vi "Target_new.vi"() -> ()   [LabVIEW 2013]
uses:
  <vilib>/Platform/TimedLoop/XDataNode/timing_clust.ctl
  <vilib>/Platform/TimedLoop/XDataNode/nitl_modes.ctl
  <vilib>/Platform/TimedLoop/XDataNode/wakeup.ctl
  <vilib>/rvi/Emulation/niFpgaSctlEmulationGetInTimedLoop.vi
  <vilib>/rvi/Emulation/niFpgaEmulationReportErrorSimple.vi
  <vilib>/rvi/Emulation/niFpgaGetClockAttributes.vi
  <vilib>/rvi/Emulation/niFpgaCriticalErrorInLSC.vi
  <vilib>/rvi/interface/RandomDataEmulation/nirviRandomDataFPGAFIFO.vi
  <vilib>/rvi/interface/RandomDataEmulation/niFpgaRandomDataHandleErrors.vi
  <vilib>/rvi/DataTransferAndStorage/Container/Common/niFpgaContainerGetUniqueNameForEmu.vi
  <vilib>/rvi/Memory/Memory_Emulation/niFpgaMemoryEmulationReadFromVariant.vi
  <vilib>/rvi/Memory/Memory_Emulation/niFpgaMemoryFastEmulationDramWriteAndRequestData.vi
  <vilib>/rvi/Memory/Memory_Emulation/niFpgaMemoryEmulationDramWriteAndRequestData.vi
  <vilib>/rvi/Memory/Memory_Emulation/niFpgaMemoryEmulationWriteToVariant.vi
  <vilib>/Platform/TimedLoop/XDataNode/XDataNode.xnode
  <vilib>/rvi/DataTransferAndStorage/Container/XNode/niFpgaContainer.xnode
  <vilib>/rvi/interface/RandomDataEmulation/nirviRandomDataFpgaReadWriteTemplate.vi
  <vilib>/rvi/Memory/Memory_Emulation/niFpgaMemoryEmulationDramRetrieveData.vi
  <vilib>/Platform/TimedLoop/XDataNode/XDNodeRunTimeDep.lvlib
panel:
  out "Записали FIFO":bool
  in  "Кон_адр":u32
  in  "FIFO":bool
  in  "Address":u32
  out "Data":u8
  in  "4":u8=4
  in  "2":u8=2
  out "Number of Elements to Write":u32
  in  "Чтение DRAM":bool
  in  "Нач_адр":u32
  in  "HOST":bool
  in  "D-0":u32
  in  "Запись в DRAM":bool
  in  "Стоп":bool
  in  "2097152":u32=2146304
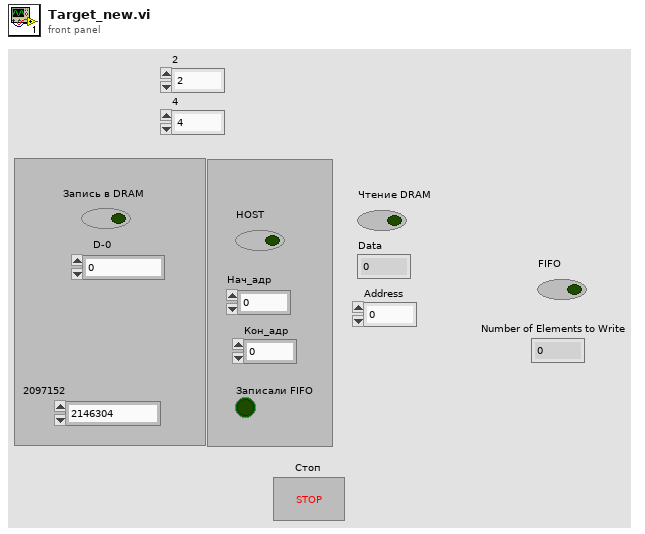
[diagram p1: front panel]
types:
  T1 = typedef "XDNodeRunTimeDep.lvlib/timing_clust.ctl" = cluster{"Expected End [f-1]":u64, "Actual End [f-1]":u64, "Finished Late? [f-1]":bool, "Expected End [i-1]":u64, "Actual End [i-1]":u64, "Finished Late? [i-1]":bool, "Expected Start [i]":u64, "Actual Start [i]":u64, "Expected Start [f]":u64, "Actual Start [f]":u64, "Source Name":string, "Structure Name":string, "Period":i64, "Deadline":i64, "Offset":i64, "Start":i64, "Priority":i32, "Timeout":i32, "Mode":T2, "Wakeup Reason":T3, "Error":errorcluster, "Source Type":string, "Secondary Source Type":string, "Global End Time":u64, "Global Start Time":u64, "Frame Duration":u64, "Iteration Duration":u64, "Assigned CPU":i32, "I/O Scan Engine Mode":u32}
  T2 = typedef "XDNodeRunTimeDep.lvlib/nitl_modes.ctl" = enum32{"No Change", "Process missed periods, maintain original phase", "Discard missed periods, maintain original phase", "Process missed periods, ignore original phase", "Discard missed periods, ignore original phase"}
  T3 = typedef "XDNodeRunTimeDep.lvlib/wakeup.ctl" = enum32{"Normal", "Aborted", "Asynchronous wakeup", "Timing source error", "Timed loop error", "Timeout"}
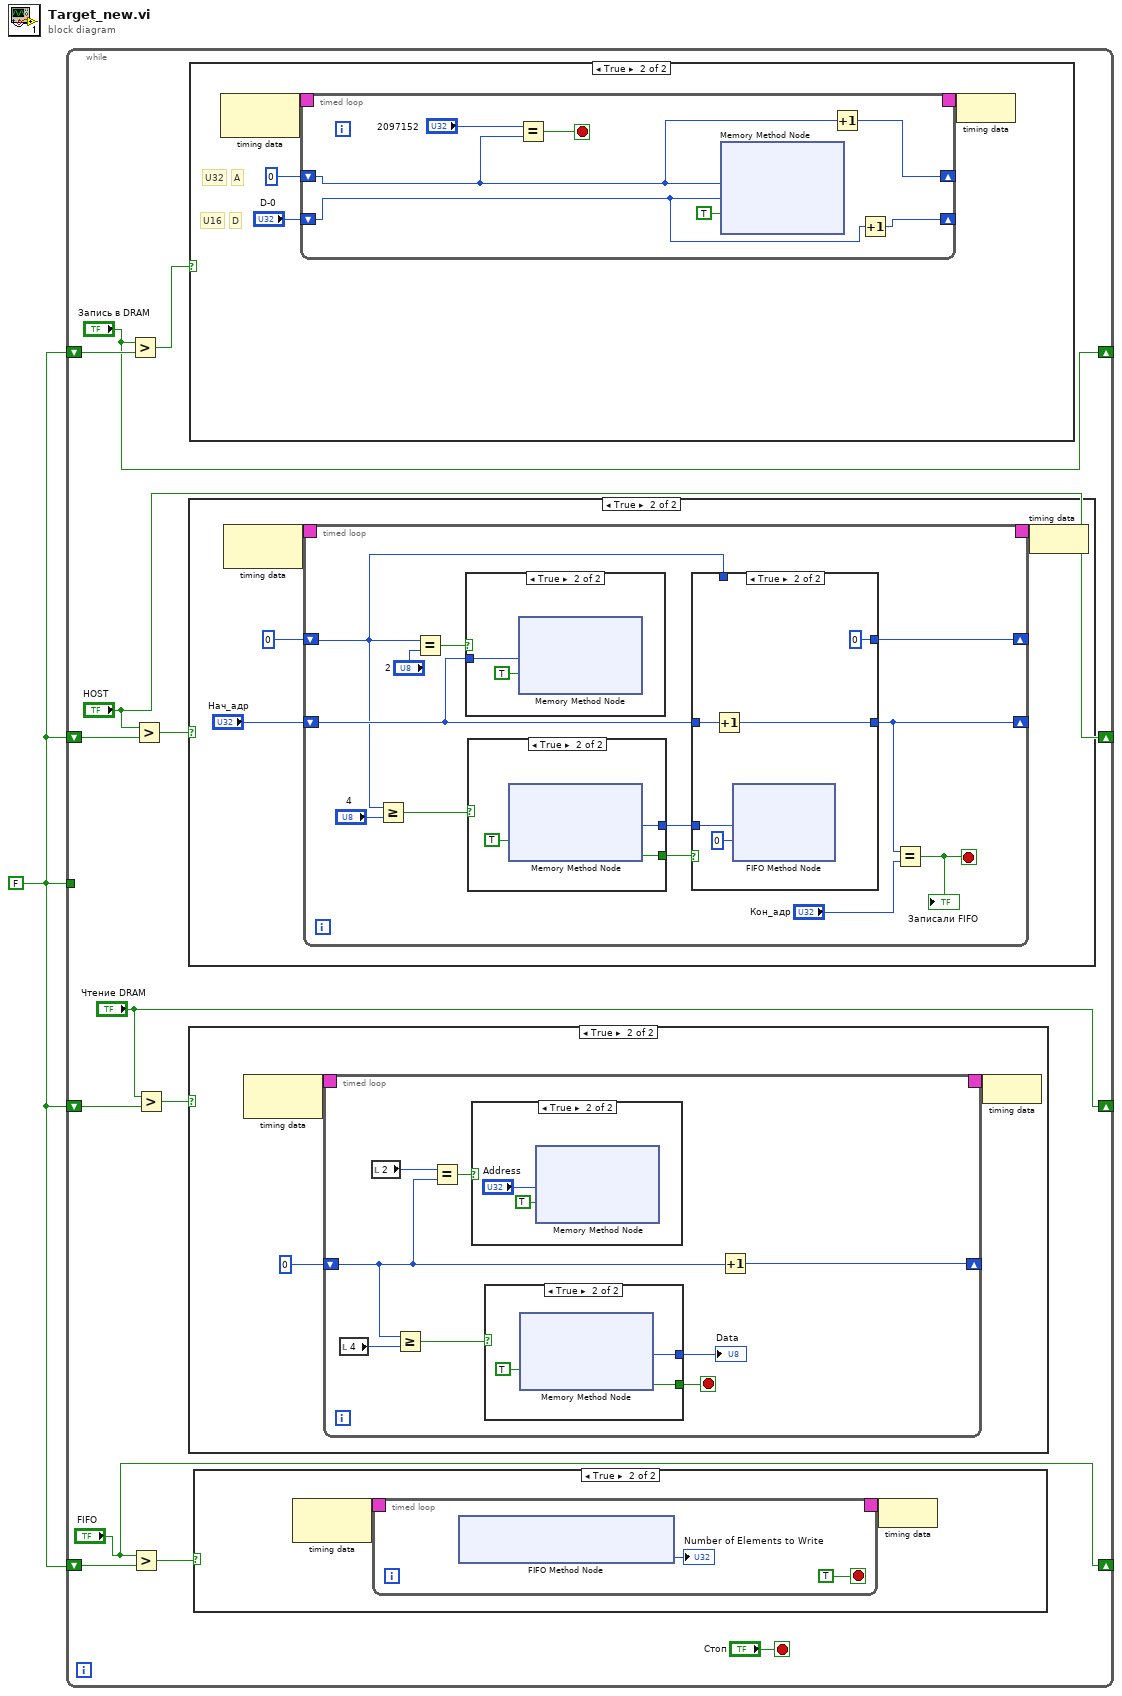
[diagram p0: block diagram]
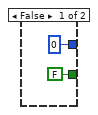
[diagram p4: hidden frame]
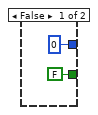
[diagram p7: hidden frame]
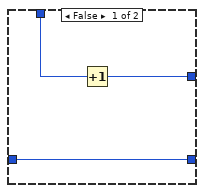
[diagram p9: hidden frame]
diagram:
  w1 = FALSE
  n1 = while {
    shift-right: ["Запись в DRAM"] -> _
    shift-left: w1 -> [w14]
    shift-right: ["HOST"] -> _
    shift-left: w1 -> [w10]
    shift-right: ["Чтение DRAM"] -> _
    shift-left: w1 -> [w8]
    shift-right: ["FIFO"] -> _
    shift-left: w1 -> [w5]
    tunnel: w1 -> [_]
    stop <- "Стоп" stop-if-true
    n2 = Greater?(x="Запись в DRAM", y=w14) -> (0:w12:bool)
    n3 = Greater?(x="FIFO", y=w5) -> (0:w4:bool)
    n4 = Greater?(x="HOST", y=w10) -> (0:w11:bool)
    n5 = Greater?(x="Чтение DRAM", y=w8) -> (0:w6:bool)
    n6 = case shown="True" w11 {
      frame False {
      }
      frame True {
        n7 = node-c288() -> (w48:T1)  [unwired: 1 in]
        n8 = timed-loop {
          shift-right: [w59] -> _
          shift-left: "Нач_адр" -> [w53]
          timing: w48 -> [_]
          timing-out: [_] -> w47
          shift-right: [w50] -> _
          shift-left: u8 0 -> [w51]
          stop <- w60 stop-if-true
          n9 = Greater Or Equal?(x=w51, y="4") -> (x >= y?=w54:bool)
          n10 = Equal?(x=w51, y="2") -> (x = y?=w57:bool)
          n11 = case shown="True" w57 {
            tunnel: w53 -> [_ w66]
            frame False {
            }
            frame True {
              n12 = xnode ("Memory Method Node")("Address"=w66, "Input Valid"=TRUE) -> ()  [unwired: 1 in, 2 out]
            }
          }
          n13 = case shown="True" w54 {
            tunnel: [u8 0 ("Data") w64] -> w58
            tunnel: [FALSE ("Output Valid") w63] -> w52
            frame False {
            }
            frame True {
              n14 = xnode ("Memory Method Node")("Ready For Output"=TRUE) -> ("Data"=w64:u32, "Output Valid"=w63:bool)  [unwired: 1 in, 1 out]
            }
          }
          n15 = case shown="True" w52 {
            tunnel: [w68 w75] -> w59
            tunnel: w58 -> [_ w73]
            tunnel: w53 -> [w68 w72]
            tunnel: w51 -> [w70 _]
            tunnel: [w69 u8 0] -> w50
            frame False {
              n16 = Increment(x=w70) -> (x+1=w69:u8)
            }
            frame True {
              n17 = Increment(x=w72) -> (x+1=w75:u32)
              n18 = xnode ("FIFO Method Node")("Element"=w73, "Timeout"=0) -> ()  [unwired: 1 in, 2 out]
            }
          }
          n19 = Equal?(x=w59, y="Кон_адр") -> (x = y?=w60:bool)
          "Записали FIFO" <- w60
        }
        n20 = node-c288(w47) -> ()
      }
    }
    n21 = case shown="True" w6 {
      frame False {
      }
      frame True {
        n22 = node-c288() -> (w25:T1)  [unwired: 1 in]
        n23 = timed-loop {
          timing: w25 -> [_]
          timing-out: [_] -> w24
          shift-right: [w31] -> _
          shift-left: u8 0 -> [w29]
          stop <- w26 stop-if-true
          n24 = local read "4"() -> (w28:u8)
          n25 = local read "2"() -> (w30:u8)
          n26 = Greater Or Equal?(x=w29, y=w28) -> (x >= y?=w33:bool)
          n27 = Equal?(x=w30, y=w29) -> (x = y?=w32:bool)
          n28 = case shown="True" w32 {
            frame False {
            }
            frame True {
              n29 = xnode ("Memory Method Node")("Address"="Address", "Input Valid"=TRUE) -> ()  [unwired: 1 in, 2 out]
            }
          }
          n30 = case shown="True" w33 {
            tunnel: [u8 0 ("Data") w37] -> w27
            tunnel: [FALSE ("Output Valid") w36] -> w26
            frame False {
            }
            frame True {
              n31 = xnode ("Memory Method Node")("Ready For Output"=TRUE) -> ("Data"=w37:u32, "Output Valid"=w36:bool)  [unwired: 1 in, 1 out]
            }
          }
          "Data" <- w27
          n32 = Increment(x=w29) -> (x+1=w31:u8)
        }
        n33 = node-c288(w24) -> ()
      }
    }
    n34 = case shown="True" w12 {
      frame False {
      }
      frame True {
        # "D"
        # "A"
        # "U32"
        # "U16"
        n35 = node-c288() -> (w83:T1)  [unwired: 1 in]
        n36 = timed-loop {
          timing: w83 -> [_]
          timing-out: [_] -> w82
          shift-right: [w86] -> _
          shift-left: "D-0" -> [w87]
          shift-right: [w84] -> _
          shift-left: u32 0 -> [w85]
          stop <- w89 stop-if-true
          n37 = Equal?(x="2097152", y=w85) -> (x = y?=w89:bool)
          n38 = xnode ("Memory Method Node")("Address"=w85, "Data"=w87, "Input Valid"=TRUE) -> ()  [unwired: 1 in, 2 out]
          n39 = Increment(x=w85) -> (x+1=w84:u32)
          n40 = Increment(x=w87) -> (x+1=w86:u32)
        }
        n41 = node-c288(w82) -> ()
      }
    }
    n42 = case shown="True" w4 {
      frame False {
      }
      frame True {
        n43 = node-c288() -> (w16:T1)  [unwired: 1 in]
        n44 = timed-loop {
          timing: w16 -> [_]
          timing-out: [_] -> w15
          stop <- TRUE stop-if-true
          n45 = xnode ("FIFO Method Node")() -> ("Number of Elements to Write"=→"Number of Elements to Write":u32)  [unwired: 1 in, 1 out]
        }
        n46 = node-c288(w15) -> ()
      }
    }
  }
